vi "Build Response Message.vi"(8 "error in (no error)":errorcluster, 10 "Result content":string, 11 "message id in":i32) -> (0 "error out":errorcluster, 3 "MCP message out":string)   [LabVIEW 2025, in "MCP Server.lvlib"]
doc: "This VI build a JSON container with a field \"jsonrpc\" set to \"2.0\", id set to the number id, and \"result\" set to whatever content is entered."
uses:
  MCP Server.lvlib
  aaa441bb-6e8c-4ec0-8711-827d95f5656f.vi
  e71c233f-4ea6-4aba-9a41-f999e1cb3491.vi
  <vilib>/JDP Science/JSONtext/Variant to JSON Text.vi
  <vilib>/JDP Science/JSONtext/support/Format JSON Object.vi
  <vilib>/JDP Science/JSONtext/LVClass Serializer/JSONtext LVClass Serializer.lvclass
  <vilib>/JDP Science/JSONtext/JSONtext.lvlib
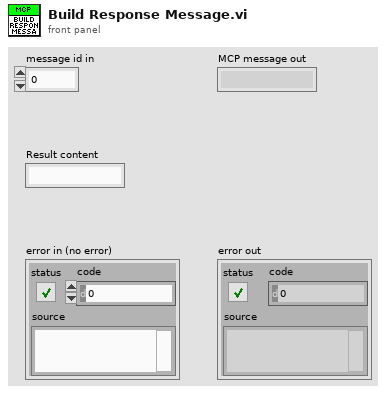
[diagram p1: front panel]
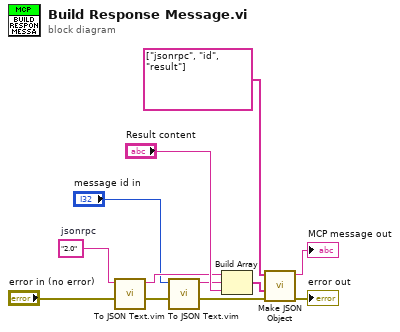
[diagram p0: block diagram]
diagram:
  w5 = "2.0"  # jsonrpc
  n1 = call "To JSON Text.vim"("error in (no error)"="error in (no error)", "Anything"=w5) -> ("error out"=w2:errorcluster, "<JSON>"=w6:string)  [unwired: 8 in]
  n2 = call "To JSON Text.vim"("error in (no error)"=w2, "Anything"="message id in") -> ("error out"=w1:errorcluster, "<JSON>"=w4:string)  [unwired: 8 in]
  n3 = Build Array(w6, w4, "Result content") -> (w7:string[])
  n4 = call <vilib>:"Make JSON Object.vi"("error in (no error)"=w1, "JSON Items"=w7, "Item Names"=string[] ["jsonrpc", "id", "result"]) -> ("error out"=→"error out":errorcluster, "<JSON>"=→"MCP message out":string)  [unwired: 7 in]
